vi "Wait Until Done.vi"(8 "error in (no error)":errorcluster, 11 "VISA resource name":refnum<visa-resource-name>) -> (0 "error out":errorcluster, 3 "VISA resource name out":refnum<visa-resource-name>)   [LabVIEW 2019, in "SpectraPro.lvlib"]
uses:
  SpectraPro.lvlib
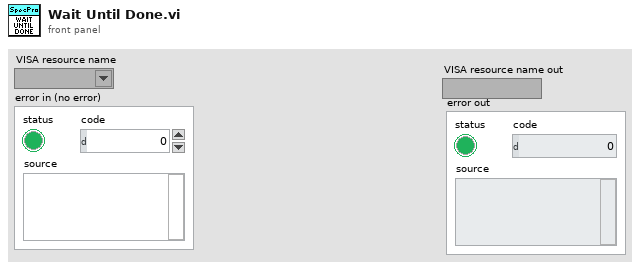
[diagram p1: front panel]
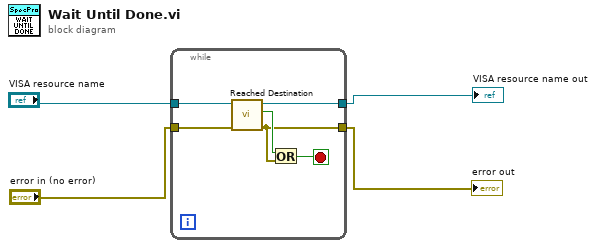
[diagram p0: block diagram]
diagram:
  n1 = while {
    tunnel: "VISA resource name" -> [w10]
    tunnel: [w9] -> w3
    tunnel: "error in (no error)" -> [w8]
    tunnel: [w5] -> w1
    stop <- w7 stop-if-true
    n2 = call "Reached Destination.vi"("error in (no error)"=w8, "VISA resource name"=w10) -> ("error out"=w5:errorcluster, "Done"=w6:bool, "VISA resource name out"=w9:refnum<visa-resource-name>)  [unwired: 6 in, 1 out]
    n3 = Or(x=w6, y=w5) -> (x .or. y?=w7:bool)
  }
  "VISA resource name out" <- w3
  "error out" <- w1
